vi "Array-Rotate and Insert.vi"(0 "Array in":dbl[](array[numeric]), 7 "Value":dbl) -> (4 "Array out":dbl[](array[numeric]))   [LabVIEW 2020]
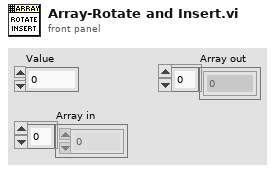
[diagram p1: front panel]
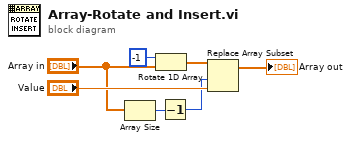
[diagram p0: block diagram]
diagram:
  n1 = Array Size(array="Array in") -> (size(s)=w2:i32)
  n2 = Rotate 1D Array(1:"Array in", 2:-1 ("n")) -> (0:w4:dbl[])
  n3 = Decrement(x=w2) -> (x-1=w6:i32)
  n4 = Replace Array Subset(array=w4, new element="Value", index=w6) -> (→"Array out":dbl[])
